vi "Request Data JSON.vi"(8 "error in (no error)":errorcluster, 11 "BatchRequest in":refnum<class "BatchRequest.lvclass">) -> (0 "error out":errorcluster, 2 "Request Data JSON":string, 3 "BatchRequest out":refnum<class "BatchRequest.lvclass">)   [LabVIEW 2020, in "obs-websocket.lvlib" / "BatchRequest.lvclass"]
uses:
  BatchRequest.lvclass
  C:/dev/lv20CE/lv-obs-websocket/obs-websocket/Request/Request.lvclass
  BatchRequest.lvclass/BatchRequest.ctl
  c1d0a5ec-5f0d-4105-80b5-21fd02b79280.vi
  bb4bdc54-ba85-4725-80f8-e87ea2ffd2d3.vi
  ffdde1ae-33fa-4b09-a2b9-8adc178e6498.vi
  <vilib>/JDP Science/JSONtext/Variant to JSON Text.vi
  <vilib>/JDP Science/JSONtext/support/Format JSON Array Text.vi
  <vilib>/JDP Science/JSONtext/LVClass Serializer/JSONtext LVClass Serializer.lvclass
  Request/Request.lvclass
  <vilib>/JDP Science/JSONtext/JSONtext.lvlib
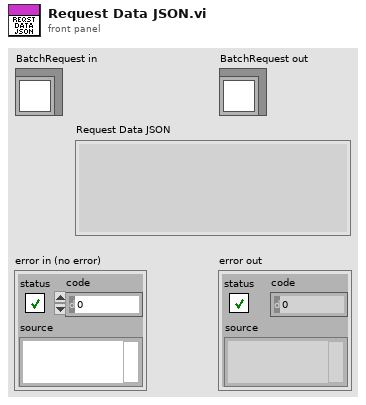
[diagram p1: front panel]
types:
  T1 = typedef "obs-websocket.lvlib/Batch Execution Type.ctl" = i16
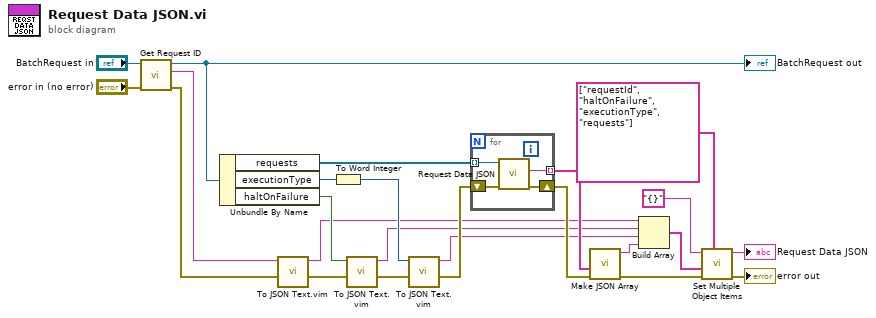
[diagram p0: block diagram]
diagram:
  n1 = call "Get Request ID.vi"("error in (no error)"="error in (no error)", "Request in"="BatchRequest in") -> ("error out"=w17:errorcluster, "Request ID"=w18:string, "Request out"=w5:refnum<class "BatchRequest.lvclass">)  [unwired: 7 in]
  "BatchRequest out" <- w5
  n2 = Unbundle By Name(w5) -> ("requests"=w2:refnum<class "Request.lvclass">[], "executionType"=w3:T1, "haltOnFailure"=w4:bool)
  n3 = call "To JSON Text.vim"("error in (no error)"=w17, "Anything"=w18) -> ("error out"=w22:errorcluster, "<JSON>"=w1:string)  [unwired: 8 in]
  n4 = To Word Integer(number=w3) -> (16bit integer=w15:T1)
  n5 = call "To JSON Text.vim"("error in (no error)"=w22, "Anything"=w4) -> ("error out"=w16:errorcluster, "<JSON>"=w14:string)  [unwired: 8 in]
  n6 = call "To JSON Text.vim"("error in (no error)"=w16, "Anything"=w15) -> ("error out"=w23:errorcluster, "<JSON>"=w13:string)  [unwired: 8 in]
  n7 = for {
    tunnel: w2 -> [w28] mode=indexing
    tunnel: [w27] -> w19 mode=indexing
    shift-right: [w26] -> w24
    shift-left: w23 -> [w25]
    n8 = call-dynamic "Request Data JSON.vi"("error in (no error)"=w25, "Request in"=w28) -> ("error out"=w26:errorcluster, "Request Data JSON"=w27:string)  [unwired: 7 in, 1 out]
  }
  n9 = call <vilib>:"Make JSON Array.vi"("error in (no error)"=w24, "JSON Elements"=w19) -> ("error out"=w10:errorcluster, "<JSON>"=w12:string)  [unwired: 8 in]
  n10 = Build Array(w1, w14, w13, w12) -> (w11:string[])
  n11 = call <vilib>:"Set Multiple Object Items.vi"("Item Names"=string[] ["requestId", "haltOnFailure", "executionType", "requests"], "error in (no error)"=w10, "JSON Items"=w11, "JSON"="{}") -> ("error out"=→"error out":errorcluster, "<JSON>"=→"Request Data JSON":string)  [unwired: 5 in]
